vi "生成文件校验码.vi"() -> ()   [LabVIEW 2017]
uses:
  <vilib>/Utility/sysdir.llb/System Directory Type.ctl
panel:
  out "MD5 message-digest 3":string caption="MD5信息摘要"
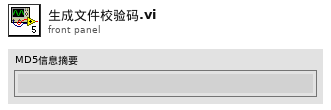
[diagram p1: front panel]
types:
  T1 = typedef "System Directory Type.ctl" = i32
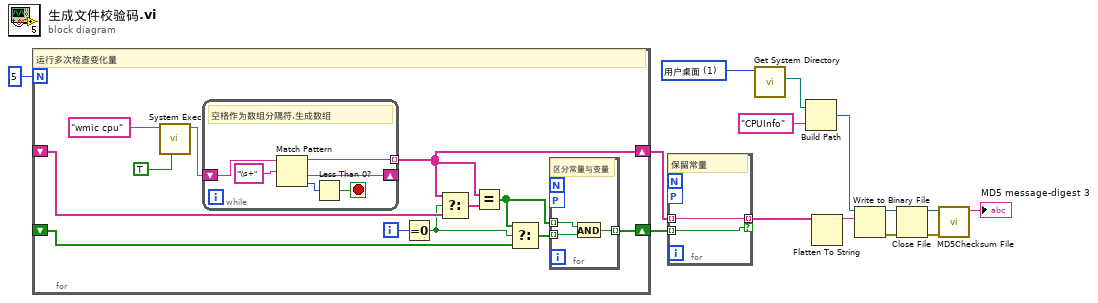
[diagram p0: block diagram]
diagram:
  w5 = T1 1 items=["用户目录"=0, "用户桌面"=1, "用户文档"=2, "用户应用程序数据"=3, "用户设置"=4, "用户临时目录"=5, "公共文档"=6, "公共应用程序数据"=7, "公共设置"=8, "公共缓存"=13, "系统核心库"=9, "系统安装库"=10, "应用程序文件"=11, "启动盘根目录"=12] ("system directory type")
  n1 = for {
    N: 5 -> [_]
    shift-right: [w16] -> w8
    shift-left: _ -> [w22]
    shift-right: [w21] -> w6
    shift-left: _ -> [w19]
    i -> [w24]
    # "运行多次检查变化量"
    n2 = call <vilib>:"System Exec.vi"("run minimized? (F)"=TRUE, "command line"="wmic cpu") -> ("standard output"=w25:string)  [unwired: 6 in, 3 out]
    n3 = while {
      shift-right: [w30] -> _
      shift-left: w25 -> [w35]
      tunnel: [w33] -> w16 mode=indexing
      stop <- w31 stop-if-true
      # "空格作为数组分隔符,生成数组"
      n4 = Match Pattern(string=w35, regular expression="\\s+" ("正则表达式")) -> (before substring=w33:string, after substring=w30:string, offset past match=w32:i32)  [unwired: 1 in, 1 out]
      n5 = Less Than 0?(x=w32) -> (x < 0?=w31:bool)
    }
    n6 = Equal To 0?(x=w24) -> (x = 0?=w20:bool)
    n7 = Select(t=w16, s=w20, f=w22) -> (s? t:f=w23:string[])
    n8 = Equal?(x=w16, y=w23) -> (x = y?=w15:bool[])
    n9 = Select(t=w15, s=w20, f=w19) -> (s? t:f=w18:bool[])
    n10 = for {
      tunnel: w15 -> [w29] mode=indexing
      tunnel: [w28] -> w21 mode=indexing
      tunnel: w18 -> [w27] mode=indexing
      workers-P: _ -> [_]
      # "区分常量与变量"
      n11 = And(x=w29, y=w27) -> (x .and. y?=w28:bool)
    }
  }
  n12 = for {
    tunnel: w8 -> [w37] mode=indexing
    tunnel: w6 -> [w36] mode=indexing
    tunnel: [w37] -> w7 mode=indexing if=w36
    workers-P: _ -> [_]
    # "保留常量"
  }
  n13 = call <vilib>:"Get System Directory.vi"("system directory type"=w5) -> ("system directory"=w2:path)  [unwired: 10 in]
  n14 = Build Path(base path=w2, name or relative path="CPUInfo" ("文件（使用对话框）")) -> (appended path=w4:path)
  n15 = Flatten To String(anything=w7) -> (data string=w9:string)  [unwired: 3 in, 2 out]
  n16 = Write to Binary File(file (use dialog)=w4, data=w9) -> (refnum out=w11:refnum<file>, error out=w10:errorcluster)  [unwired: 4 in, 1 out]
  n17 = Close File(refnum=w11, error in=w10) -> (path=w12:path, error out=w1:errorcluster)
  n18 = call <vilib>:"MD5Checksum File.vi"("error in (no error)"=w1, "Path"=w12) -> ("MD5 message-digest"=→"MD5 message-digest 3":string)  [unwired: 8 in, 1 out]
